vi "Serial_Write_Read_concat_Labview_xbox.vi"() -> ()   [LabVIEW 2023]
uses:
  <vilib>/MakerHub/Xbox-One-Controller/Private/Type Defs/Indicators/All Axis Data.ctl
  <vilib>/MakerHub/Xbox-One-Controller/Private/Type Defs/Indicators/DPad Enum.ctl
  <vilib>/MakerHub/Xbox-One-Controller/Public/Open First Controller.vi
  <vilib>/Instr/_visa.llb/VISA Configure Serial Port (Instr).vi
  <vilib>/MakerHub/Xbox-One-Controller/LMH-Xbox-One-Controller.lvlib
panel:
  out "All Axis":T1
  in  "Stop Button":bool
  out "Event Log":string[](array[string])
  out "error out":errorcluster
  in  "error in (no error)":errorcluster
  in  "byte count\nRead":u32
  in  "Number 2":u32
  in  "Number 1":u32
  in  "Loop Timer":u32
  out "Concatenated \nNumber":string
  in  "baud rate (9600)":u32=9600
  in  "VISA resource name":refnum<visa-resource-name>
  in  "stop":bool
  out "byte count Sent":u32
  out "read buffer":string
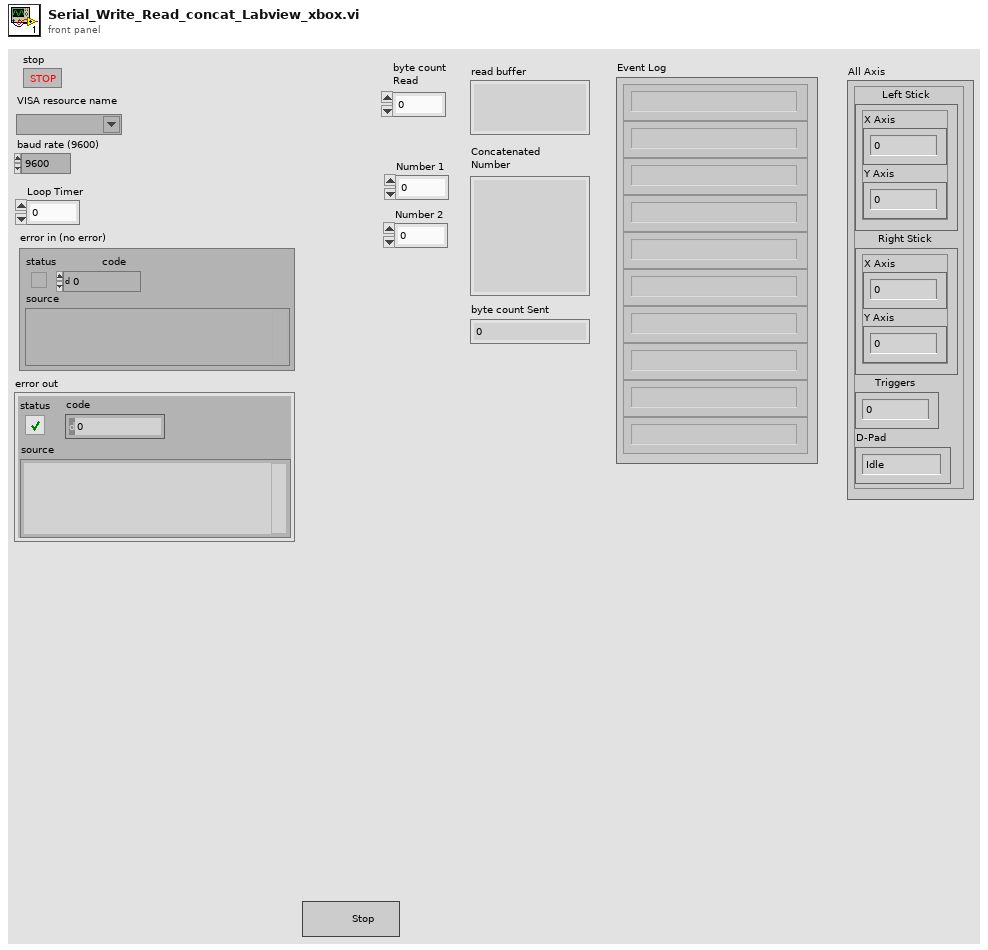
[diagram p1: front panel]
types:
  T1 = typedef "LMH-Xbox-One-Controller.lvlib/All Axis Data.ctl" = cluster{"Left Stick":cluster{"X Axis":i32, "Y Axis":i32}, "Right Stick":cluster{"X Axis":i32, "Y Axis":i32}, "Triggers":i32, "D-Pad":T2}
  T2 = typedef "LMH-Xbox-One-Controller.lvlib/DPad Enum.ctl" = enum16{"Idle", "Up", "Up / Right", "Right", "Down / Right", "Down", "Down / Left", "Left", "Up / Left"}
  T3 = typedef "LMH-Xbox-One-Controller.lvlib/Xbox One Controller Ref.ctl" = cluster{"Controller Ref":refnum<k1>, "Event Refnum":refnum<event-registration>, "Worker Ref":refnum<vi>}
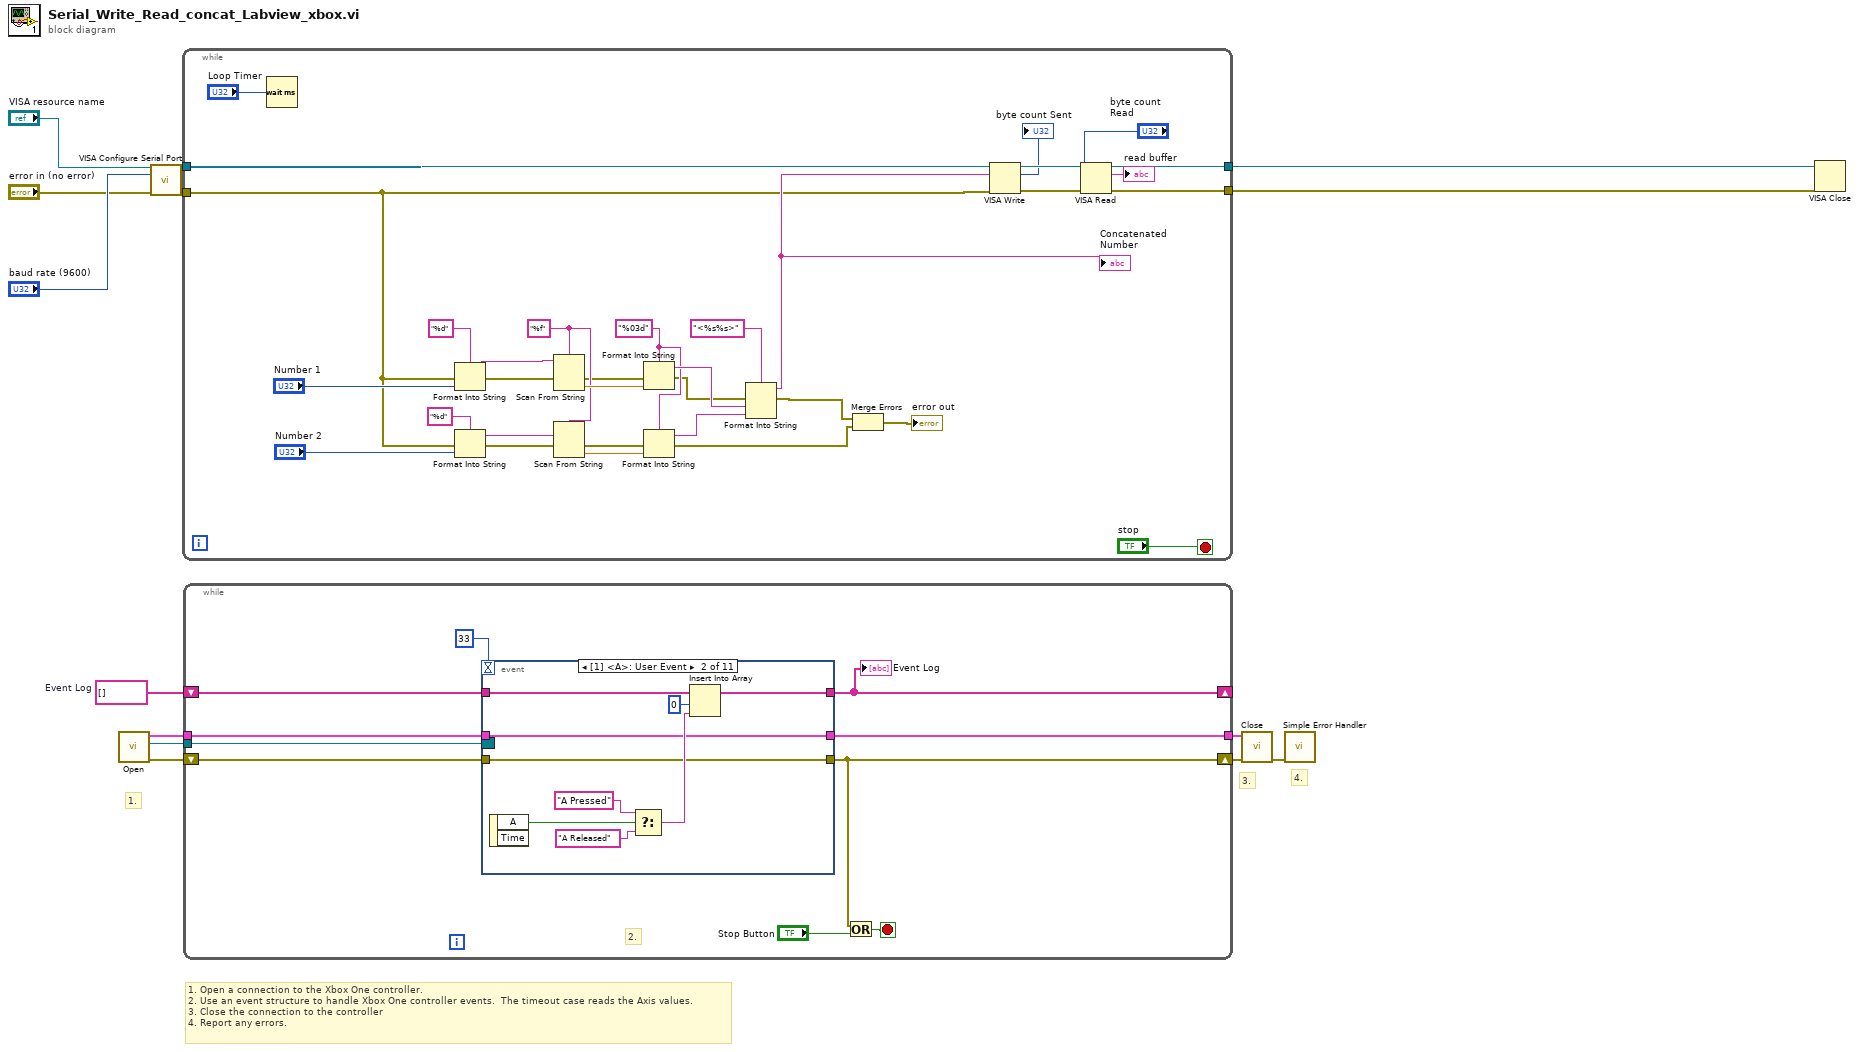
[diagram p0: block diagram]
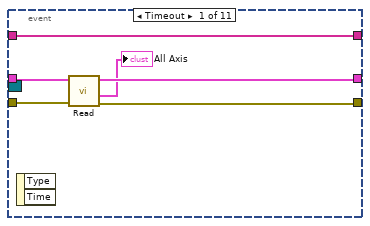
[diagram p2: hidden frame]
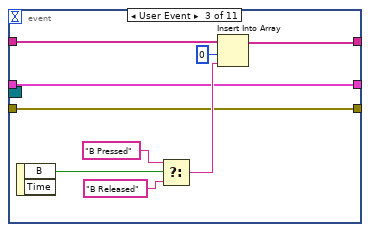
[diagram p3: hidden frame]
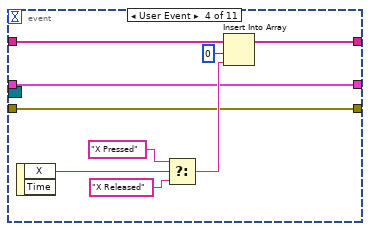
[diagram p4: hidden frame]
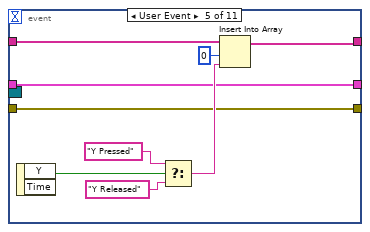
[diagram p5: hidden frame]
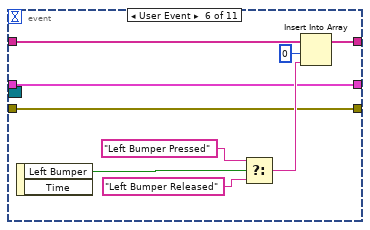
[diagram p6: hidden frame]
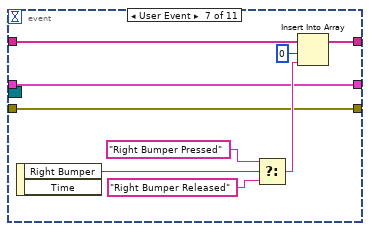
[diagram p7: hidden frame]
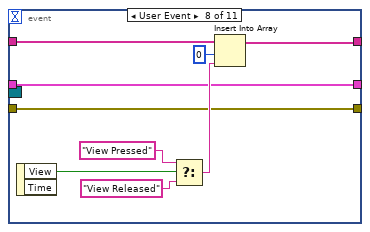
[diagram p8: hidden frame]
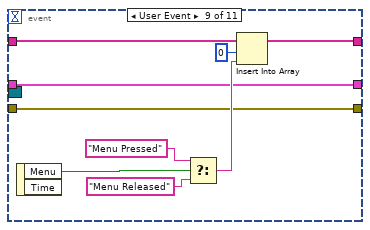
[diagram p9: hidden frame]
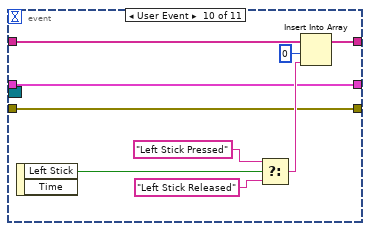
[diagram p10: hidden frame]
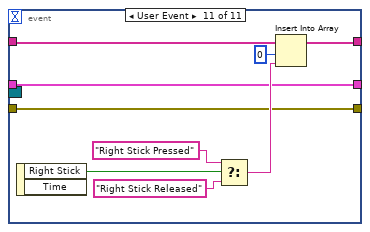
[diagram p11: hidden frame]
diagram:
  w2 = string[] []  # Event Log
  # "1. Open a connection to the Xbox One controller.\n2. Use an event structure to handle Xbox One controller events.  The timeout case reads the Axis values.\n3. Close the connection to the controller\n4. Report any errors."
  # "4."
  # "3."
  # "1."
  n1 = call-poly <vilib>:"Open.vi"() -> ("Error Out"=w5:errorcluster, "Event Refnum"=w4:refnum<event-registration>, "Xbox One Controller"=w3:T3)  [unwired: 9 in]
  n2 = call-poly "VISA Configure Serial Port"("VISA resource name"="VISA resource name", "baud rate (9600)"="baud rate (9600)", "error in (no error)"="error in (no error)") -> ("VISA resource name out"=w12:refnum<visa-resource-name>, "error out"=w11:errorcluster)  [unwired: 11 in]
  n3 = while {
    tunnel: [w46] -> w14
    tunnel: [w44] -> w13
    tunnel: w12 -> [w41]
    tunnel: w11 -> [w18]
    stop <- "stop" stop-if-true
    w30 = "%f" ("format string")
    w32 = "%03d" ("format string")
    n4 = Wait (ms)(milliseconds to wait="Loop Timer") -> ()  [unwired: 1 out]
    n5 = Format Into String(format string="%d", error in=w18, "Number 1") -> (resulting string=w36:string, error out=w23:errorcluster)  [unwired: 1 in]
    n6 = Format Into String(format string="%d", error in=w18, "Number 2") -> (resulting string=w31:string, error out=w20:errorcluster)  [unwired: 1 in]
    n7 = Scan From String(format string=w30, input string=w36, error in=w23) -> (error out=w22:errorcluster, output 1=w37:dbl)  [unwired: 2 in, 2 out]
    n8 = Scan From String(format string=w30, input string=w31, error in=w20) -> (error out=w19:errorcluster, output 1=w27:dbl)  [unwired: 2 in, 2 out]
    n9 = Format Into String(format string=w32, error in=w22, w37) -> (resulting string=w35:string, error out=w21:errorcluster)  [unwired: 1 in]
    n10 = Format Into String(format string=w32, error in=w19, w27) -> (resulting string=w33:string, error out=w16:errorcluster)  [unwired: 1 in]
    n11 = Format Into String(format string="<%s%s>", error in=w21, w35, w33) -> (resulting string=w26:string, error out=w17:errorcluster)  [unwired: 1 in]
    "Concatenated \nNumber" <- w26
    n12 = Merge Errors(w17, w16) -> (→"error out":errorcluster)
    n13 = VISA Write(VISA resource name=w41, write buffer=w26, error in (no error)=w18) -> (VISA resource name out=w47:refnum<visa-resource-name>, return count=→"byte count Sent":u32, error out=w43:errorcluster)
    n14 = VISA Read(VISA resource name=w47, byte count="byte count\nRead", error in (no error)=w43) -> (VISA resource name out=w46:refnum<visa-resource-name>, read buffer=→"read buffer":string, error out=w44:errorcluster)  [unwired: 1 out]
  }
  n15 = while {
    tunnel: w4 -> [w50]
    shift-right: [w53] -> w6
    shift-left: w5 -> [w56]
    tunnel: w3 -> [w57]
    tunnel: [w52] -> w7
    shift-right: [w48] -> _
    shift-left: w2 -> [w49]
    stop <- w55 stop-if-true
    # "2."
    n16 = event shown="[1] <A>: User Event" {
      selector: w50 -> [_ _ _ _ _ _ _ _ _ _ _]
      dyn-events: _ -> [_ _ _ _ _ _ _ _ _ _ _]
      timeout: 33 -> [_ _ _ _ _ _ _ _ _ _ _]
      tunnel: w57 -> [w63 w66 w74 w86 w96 w104 w111 w121 w128 w138 w148]
      tunnel: w56 -> [w62 w65 w75 w87 w95 w105 w112 w122 w129 w137 w147]
      tunnel: [w58 w65 w75 w87 w95 w105 w112 w122 w129 w137 w147] -> w53
      tunnel: [w61 w66 w74 w86 w96 w104 w111 w121 w128 w138 w148] -> w52
      tunnel: w49 -> [w59 w72 w77 w85 w93 w103 w113 w120 w131 w140 w149]
      tunnel: [w59 w67 w76 w84 w92 w102 w114 w119 w132 w141 w150] -> w48
      event Timeout {
        n17 = event-data() -> ()  [unwired: 1 in, 2 out]
        n18 = call <vilib>:"Read.vi"("Error In"=w62, "Xbox One Controller Ref"=w63) -> ("Error Out"=w58:errorcluster, "All Axis"=→"All Axis":T1, "Xbox One Controller Ref"=w61:T3)  [unwired: 6 in, 1 out]
      }
      event User Event {
        n19 = event-data() -> ("A"=w71:bool)  [unwired: 1 in, 1 out]
        n20 = Select(t="A Pressed" ("String"), s=w71, f="A Released" ("String")) -> (s? t:f=w68:string)
        n21 = Insert Into Array(array=w72, index=0, new element=w68) -> (w67:string[])
      }
      event User Event {
        n22 = event-data() -> ("B"=w78:bool)  [unwired: 1 in, 1 out]
        n23 = Select(t="B Pressed" ("String"), s=w78, f="B Released" ("String")) -> (s? t:f=w79:string)
        n24 = Insert Into Array(array=w77, index=0, new element=w79) -> (w76:string[])
      }
      event User Event {
        n25 = event-data() -> ("X"=w83:bool)  [unwired: 1 in, 1 out]
        n26 = Select(t="X Pressed" ("String"), s=w83, f="X Released" ("String")) -> (s? t:f=w88:string)
        n27 = Insert Into Array(array=w85, index=0, new element=w88) -> (w84:string[])
      }
      event User Event {
        n28 = event-data() -> ("Y"=w94:bool)  [unwired: 1 in, 1 out]
        n29 = Select(t="Y Pressed" ("String"), s=w94, f="Y Released" ("String")) -> (s? t:f=w97:string)
        n30 = Insert Into Array(array=w93, index=0, new element=w97) -> (w92:string[])
      }
      event User Event {
        n31 = event-data() -> ("Left Bumper"=w101:bool)  [unwired: 1 in, 1 out]
        n32 = Select(t="Left Bumper Pressed" ("String"), s=w101, f="Left Bumper Released" ("String")) -> (s? t:f=w106:string)
        n33 = Insert Into Array(array=w103, index=0, new element=w106) -> (w102:string[])
      }
      event User Event {
        n34 = event-data() -> ("Right Bumper"=w110:bool)  [unwired: 1 in, 1 out]
        n35 = Select(t="Right Bumper Pressed" ("String"), s=w110, f="Right Bumper Released" ("String")) -> (s? t:f=w115:string)
        n36 = Insert Into Array(array=w113, index=0, new element=w115) -> (w114:string[])
      }
      event User Event {
        n37 = event-data() -> ("View"=w123:bool)  [unwired: 1 in, 1 out]
        n38 = Select(t="View Pressed" ("String"), s=w123, f="View Released" ("String")) -> (s? t:f=w124:string)
        n39 = Insert Into Array(array=w120, index=0, new element=w124) -> (w119:string[])
      }
      event User Event {
        n40 = event-data() -> ("Menu"=w130:bool)  [unwired: 1 in, 1 out]
        n41 = Select(t="Menu Pressed" ("String"), s=w130, f="Menu Released" ("String")) -> (s? t:f=w133:string)
        n42 = Insert Into Array(array=w131, index=0, new element=w133) -> (w132:string[])
      }
      event User Event {
        n43 = event-data() -> ("Left Stick"=w139:bool)  [unwired: 1 in, 1 out]
        n44 = Select(t="Left Stick Pressed" ("String"), s=w139, f="Left Stick Released" ("String")) -> (s? t:f=w142:string)
        n45 = Insert Into Array(array=w140, index=0, new element=w142) -> (w141:string[])
      }
      event User Event {
        n46 = event-data() -> ("Right Stick"=w146:bool)  [unwired: 1 in, 1 out]
        n47 = Select(t="Right Stick Pressed" ("String"), s=w146, f="Right Stick Released" ("String")) -> (s? t:f=w151:string)
        n48 = Insert Into Array(array=w149, index=0, new element=w151) -> (w150:string[])
      }
    }
    "Event Log" <- w48
    n49 = Or(x=w53, y="Stop Button") -> (x .or. y?=w55:bool)
  }
  n50 = call <vilib>:"Close.vi"("Error In"=w6, "Xbox One Controller Ref"=w7) -> ("Error Out"=w1:errorcluster)  [unwired: 9 in]
  n51 = call <vilib>:"Simple Error Handler.vi"("error in (no error)"=w1) -> ()  [unwired: 4 in, 5 out]
  n52 = VISA Close(VISA resource name=w14, error in (no error)=w13) -> ()  [unwired: 1 out]
